vi "SysLog Interface cRIO.vi"(8 "Fehler (in)":errorcluster caption="Fehlereingang", 11 "Cluster (in)":T1={"FehlermeldungsCode"=-1, "ErfolgsmeldungsCode"=-1, "ParameterListenString"="", "intern"=FALSE}) -> (0 "Fehler (Ausgang)":errorcluster)   [LabVIEW 2020, in "SysLog_cRIO.lvlib"]
doc: "Interface zur Fehlerbehandlung cRIO\nFehler (Fehlereingang) wird in die #ErrorLogHistory aufgenommen.\nErfolgsmeldung optional - wird nur geloggt, wenn nicht leer und BedingteDeaktivierung \"ErfolgsMeldungÖLoggen == TRUE\" \nriw - 11.06.2018"
uses:
  SysLog_cRIO.lvlib
  SysLog Interface cRIO.ctl
  Allgemein/FGV Zustaende Aktionen.ctl
  Allgemein/Allgemein.lvlib
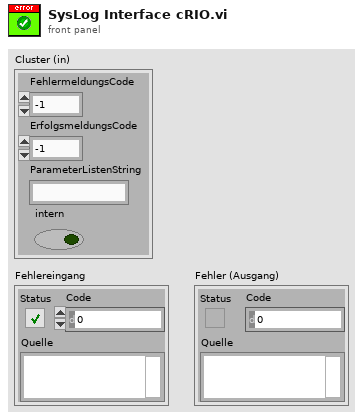
[diagram p1: front panel]
types:
  T1 = typedef "SysLog_cRIO.lvlib/SysLog Interface cRIO.ctl" = cluster{"FehlermeldungsCode":i32, "ErfolgsmeldungsCode":i32, "ParameterListenString":string, "intern":bool}
  T2 = typedef "Allgemein.lvlib/FGV Zustaende Aktionen.ctl" = enum16{"lesen", "Zustand PC", "Zustand cRIO", "Bildnummer", "Samplepoint", "Sysloglevel"}
  T3 = cluster{"SysLogLevel":u16, "Software Version":string}
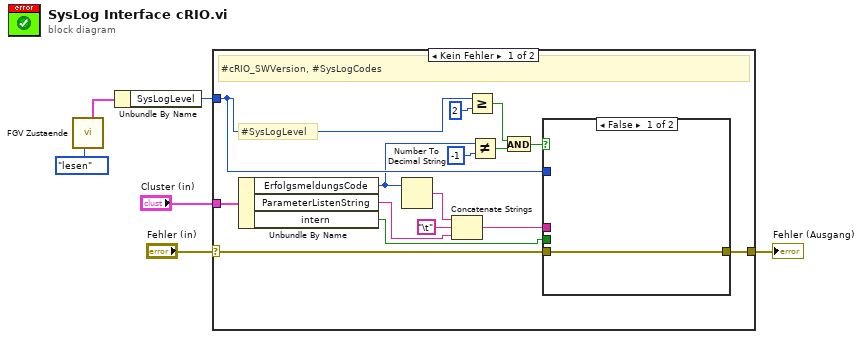
[diagram p0: block diagram]
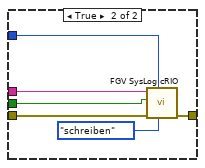
[diagram p2: hidden frame]
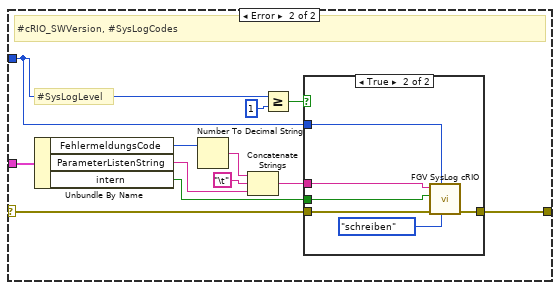
[diagram p3: hidden frame]
diagram:
  n1 = call "FGV Zustaende.vi"("Aktionen"=FGV_Zustaende_Aktionen."lesen") -> ("SL SV Cluster"=w2:T3)  [unwired: 6 in, 4 out]
  n2 = Unbundle By Name(w2) -> ("SysLogLevel"=w1:u16)
  n3 = case shown="Kein Fehler" "Fehler (in)" {
    selector: "Fehler (in)" -> [w20 w38]
    tunnel: "Cluster (in)" -> [w21 w40]
    tunnel: w1 -> [w14 w34]
    tunnel: [w15 w35] -> w3
    frame No Error {
      # "#SysLogLevel"
      # "#cRIO_SWVersion, #SysLogCodes"
      n4 = Unbundle By Name(w21) -> ("ErfolgsmeldungsCode"=w7:i32, "ParameterListenString"=w10:string, "intern"=w13:bool)
      n5 = Number To Decimal String(number=w7) -> (decimal integer string=w8:string)  [unwired: 1 in]
      n6 = Concatenate Strings(w8, "\t", w10) -> (w9:string)
      n7 = Greater Or Equal?(x=w14, y=u16 2) -> (x >= y?=w16:bool)
      n8 = Not Equal?(x=w7, y=-1) -> (x != y?=w17:bool)
      n9 = And(x=w16, y=w17) -> (x .and. y?=w18:bool)
      n10 = case shown="False" w18 {
        tunnel: w9 -> [_ w28]
        tunnel: w20 -> [w22 w27]
        tunnel: [w22 w25] -> w15
        tunnel: w14 -> [_ w24]
        tunnel: w13 -> [_ w23]
        frame False {
        }
        frame True {
          n11 = call "FGV SysLog cRIO.vi"("Aktion"=enum16{"initialisieren", "lesen", "schreiben"}."schreiben", "SysLogLevel"=w24, "Fehler (in)"=w27, "intern"=w23, "Message in"=w28) -> ("Fehler (out)"=w25:errorcluster)  [unwired: 4 in, 2 out]
        }
      }
    }
    frame Error {
      # "#SysLogLevel"
      # "#cRIO_SWVersion, #SysLogCodes"
      n12 = Unbundle By Name(w40) -> ("FehlermeldungsCode"=w30:i32, "ParameterListenString"=w39:string, "intern"=w33:bool)
      n13 = Number To Decimal String(number=w30) -> (decimal integer string=w31:string)  [unwired: 1 in]
      n14 = Concatenate Strings(w31, "\t", w39) -> (w32:string)
      n15 = Greater Or Equal?(x=w34, y=u16 1) -> (x >= y?=w36:bool)
      n16 = case shown="True" w36 {
        tunnel: w32 -> [_ w46]
        tunnel: w38 -> [w41 w45]
        tunnel: [w41 w44] -> w35
        tunnel: w34 -> [_ w43]
        tunnel: w33 -> [_ w42]
        frame False {
        }
        frame True {
          n17 = call "FGV SysLog cRIO.vi"("Aktion"=enum16{"initialisieren", "lesen", "schreiben"}."schreiben", "SysLogLevel"=w43, "Fehler (in)"=w45, "intern"=w42, "Message in"=w46) -> ("Fehler (out)"=w44:errorcluster)  [unwired: 4 in, 2 out]
        }
      }
    }
  }
  "Fehler (Ausgang)" <- w3
